vi "Init.vi"(4 "HeadDirection":T2, 6 "SnakeColor":T4={"HeadColor"=0, "BodyColor"=0, "TailColor"=0, "FeedColor"=16777224}, 7 "BG Color":u32(colorbox), 8 "error in (no error)":errorcluster, 9 "SnakeLength #BodyCells":u32, 10 "SnakeHeadPos":T3, 11 "DisplaySize":T1) -> (0 "error out":errorcluster, 3 "2D_Representer out":refnum<class "2D_Representer.lvclass">)   [LabVIEW 2018, in "2D_Representer.lvclass"]
uses:
  2D_Representer.lvclass
  Typedefs/Colors.ctl
  Typedefs/XYposition.ctl
  Typedefs/UnitDirection.ctl
  Typedefs/DisplaySize.ctl
  2D_Representer.lvclass/2D_Representer.ctl
  Snake/Snake.lvclass
  Feeder/Feeder.lvclass
panel:
  # "Connector Pane"
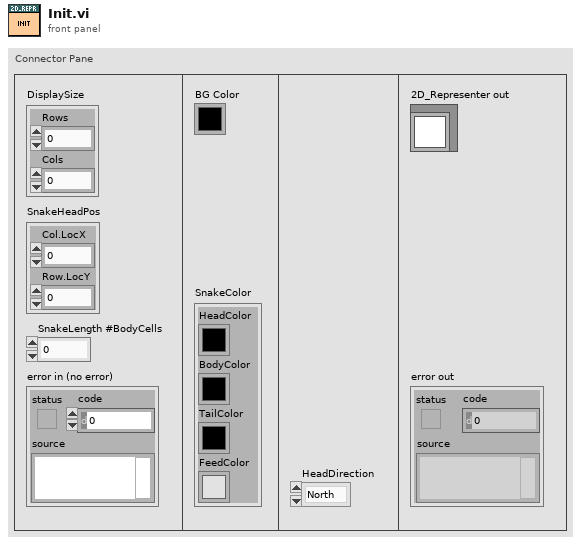
[diagram p1: front panel]
types:
  T1 = typedef "DisplaySize.ctl" = cluster{"Rows":i32, "Cols":i32}
  T2 = typedef "UnitDirection.ctl" = enum16{"North", "East", "South", "West"}
  T3 = typedef "XYposition.ctl" = cluster{"Col.LocX":i32, "Row.LocY":i32}
  T4 = typedef "Colors.ctl" = cluster{"HeadColor":u32, "BodyColor":u32, "TailColor":u32, "FeedColor":u32}
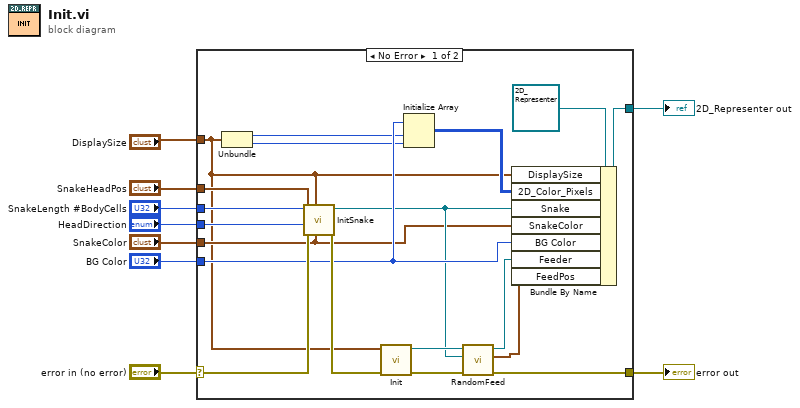
[diagram p0: block diagram]
diagram:
  n1 = case shown="No Error" "error in (no error)" {
    selector: "error in (no error)" -> [w28 w29]
    tunnel: [w16 w29] -> w8
    tunnel: [w25 _] -> w7
    tunnel: "SnakeColor" -> [w12 _]
    tunnel: "SnakeHeadPos" -> [w24 _]
    tunnel: "SnakeLength #BodyCells" -> [w23 _]
    tunnel: "BG Color" -> [w21 _]
    tunnel: "HeadDirection" -> [w22 _]
    tunnel: "DisplaySize" -> [w11 _]
    frame No Error {
      n2 = Unbundle(w11) -> ("Rows"=w20:i32, "Cols"=w19:i32)
      n3 = call "InitSnake.vi"("Colors"=w12, "DisplaySize"=w11, "error in (no error)"=w28, "HeadDirection"=w22, "HeadPos"=w24, "SnakeLength #BodyCells"=w23) -> ("error out"=w27:errorcluster, "Snake out"=w13:refnum<class "Snake.lvclass">)  [unwired: 4 in]
      n4 = call "Init.vi"("error in (no error)"=w27, "DisplaySize"=w11) -> ("error out"=w17:errorcluster, "Feeder out"=w15:refnum<class "Feeder.lvclass">)  [unwired: 8 in]
      n5 = Initialize Array(w21, w20, w19) -> (w18:u32[][])
      n6 = call "RandomFeed.vi"("error in (no error)"=w17, "Snake"=w13, "Feeder in"=w15) -> ("error out"=w16:errorcluster, "FeedPos"=w10:T3, "Feeder out"=w14:refnum<class "Feeder.lvclass">)  [unwired: 6 in]
      n7 = Bundle By Name(cluster=refnum<class "2D_Representer.lvclass"> refnum ("2D_Representer in"), "DisplaySize"=w11, "2D_Color_Pixels"=w18, "Snake"=w13, "SnakeColor"=w12, "BG Color"=w21, "Feeder"=w14, "FeedPos"=w10) -> (w25:refnum<class "2D_Representer.lvclass">)
    }
    frame Error {
    }
  }
  "error out" <- w8
  "2D_Representer out" <- w7
